vi "Init UI controls.vi"(8 "error in (no error)":errorcluster, 11 "TS UI Data in":T1) -> (0 "error out":errorcluster)   [LabVIEW 2015]
uses:
  Type defs/TS UI Data.ctl
  Type defs/Nest cluster.ctl
panel:
  # "SCANNED DATA"
  # "ITAC DATA"
  # "DoIP DATA"
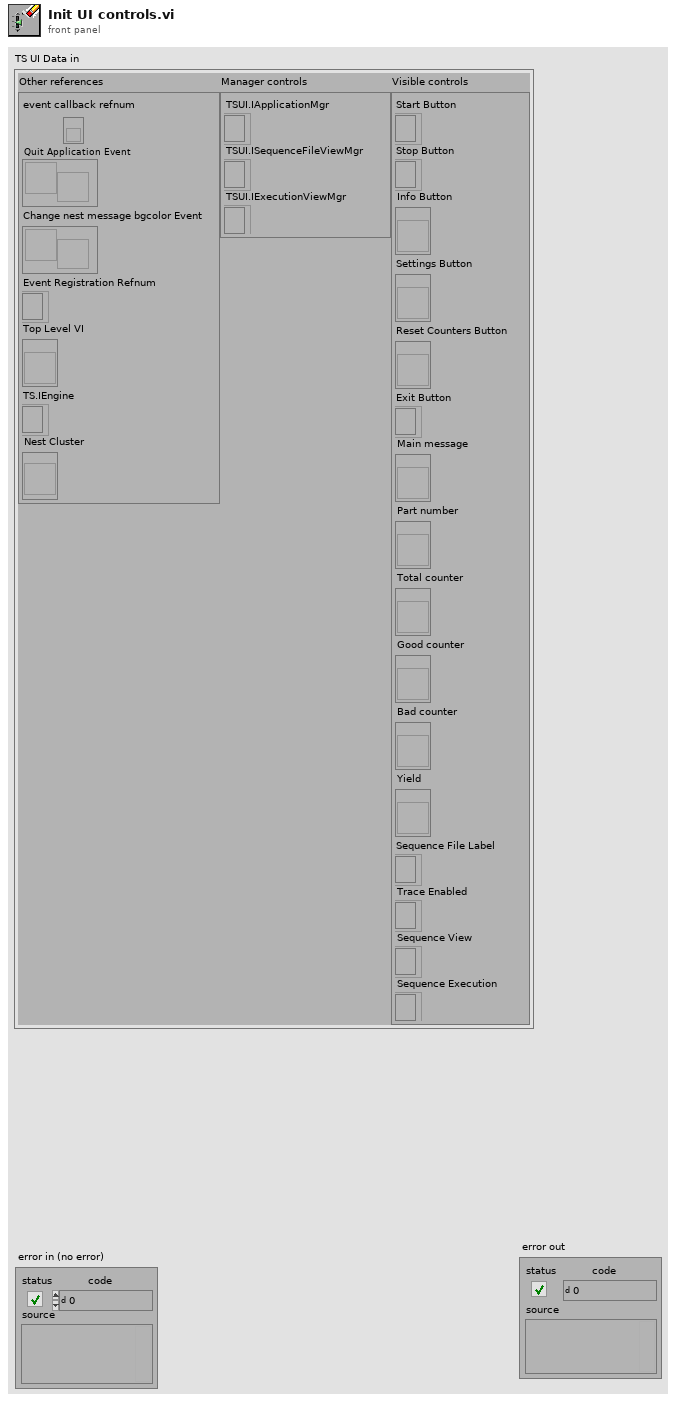
[diagram p1: front panel]
types:
  T1 = typedef "TS UI Data.ctl" = cluster{"Other references":cluster{"event callback refnum":refnum<k27>, "Quit Application Event":refnum<user-event>, "Change nest message bgcolor Event":refnum<user-event>, "event registration refnum":refnum<event-registration>, "Top Level VI":refnum<vi>, "TS.IEngine":refnum<k7>, "Nest Cluster":refnum<vi>}, "Manager controls":cluster{"TSUI.IApplicationMgr":refnum<k7>, "TSUI.ISequenceFileViewMgr":refnum<k7>, "TSUI.IExecutionViewMgr":refnum<k7>}, "Visible controls":cluster{"Start Button":refnum<k7>, "Stop Button":refnum<k7>, "Info Button":refnum<vi>, "Settings Button":refnum<vi>, "Reset Counters Button":refnum<vi>, "Exit Button":refnum<k7>, "Main message":refnum<vi>, "Part number":refnum<vi>, "Total counter":refnum<vi>, "Good counter":refnum<vi>, "Bad counter":refnum<vi>, "Yield":refnum<vi>, "Sequence File Label":refnum<k7>, "Trace Enabled":refnum<k7>, "Sequence View":refnum<k7>, "Sequence Execution":refnum<k7>}}
  T2 = enum8{"Enabled", "Disabled", "Disabled and Grayed Out"}
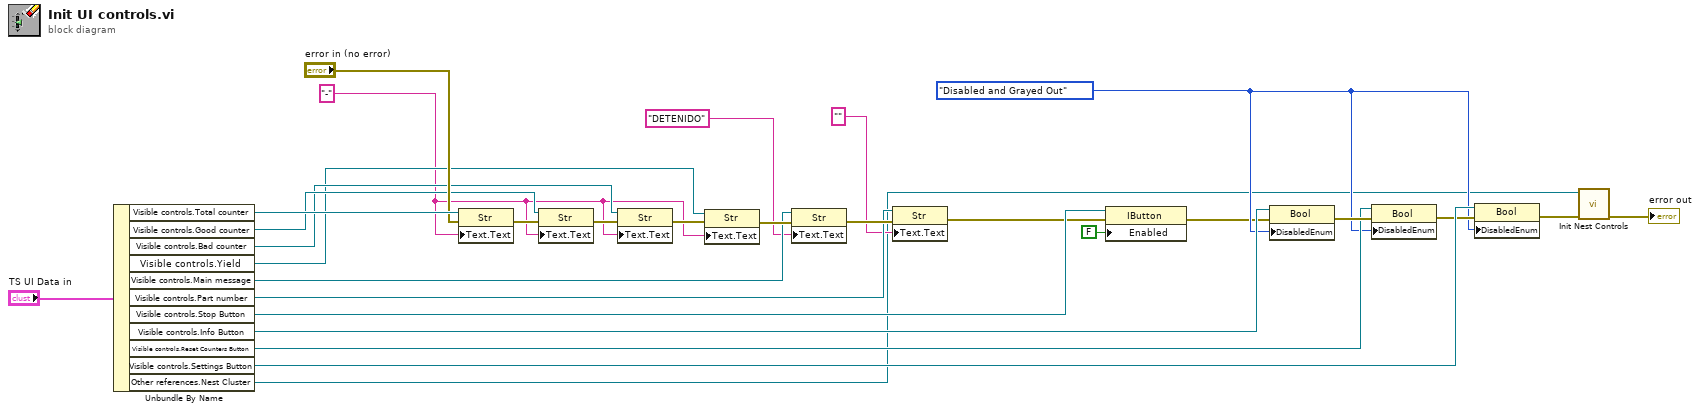
[diagram p0: block diagram]
diagram:
  w8 = T2."Disabled and Grayed Out" ("Disabled")
  w19 = "-"
  n1 = Unbundle By Name("TS UI Data in") -> ("Visible controls.Total counter"=w29:refnum<vi>, "Visible controls.Good counter"=w26:refnum<vi>, "Visible controls.Bad counter"=w24:refnum<vi>, "Visible controls.Yield"=w22:refnum<vi>, "Visible controls.Main message"=w20:refnum<vi>, "Visible controls.Part number"=w16:refnum<vi>, "Visible controls.Stop Button"=w6:refnum<k7>, "Visible controls.Info Button"=w14:refnum<vi>, "Visible controls.Reset Counters Button"=w12:refnum<vi>, "Visible controls.Settings Button"=w11:refnum<vi>, "Other references.Nest Cluster"=w3:refnum<vi>)
  n2 = property class="Str"(reference=w29, error in="error in (no error)", "Text.Text"=w19) -> (error out=w27:errorcluster)  [unwired: 1 out]
  n3 = property class="Str"(reference=w26, error in=w27, "Text.Text"=w19) -> (error out=w25:errorcluster)  [unwired: 1 out]
  n4 = property class="Str"(reference=w24, error in=w25, "Text.Text"=w19) -> (error out=w23:errorcluster)  [unwired: 1 out]
  n5 = property class="Str"(reference=w22, error in=w23, "Text.Text"=w19) -> (error out=w21:errorcluster)  [unwired: 1 out]
  n6 = property class="Str"(reference=w20, error in=w21, "Text.Text"="DETENIDO") -> (error out=w17:errorcluster)  [unwired: 1 out]
  n7 = property class="Str"(reference=w16, error in=w17, "Text.Text"="") -> (error out=w1:errorcluster)  [unwired: 1 out]
  n8 = property class="IButton"(reference=w6, error in=w1, "Enabled"=FALSE) -> (error out=w4:errorcluster)  [unwired: 1 out]
  n9 = property class="Bool"(reference=w14, error in=w4, "DisabledEnum"=w8) -> (error out=w13:errorcluster)  [unwired: 1 out]
  n10 = property class="Bool"(reference=w12, error in=w13, "DisabledEnum"=w8) -> (error out=w10:errorcluster)  [unwired: 1 out]
  n11 = property class="Bool"(reference=w11, error in=w10, "DisabledEnum"=w8) -> (error out=w7:errorcluster)  [unwired: 1 out]
  n12 = call "Init Nest Controls.vi"("error in (no error)"=w7, "Nest Cluster"=w3) -> ("error out"=→"error out":errorcluster)  [unwired: 9 in]
